vi "BRig_dataLC_Selection_PreR_Delay_l1.vi"() -> (2 "output_Selection_PreR_Delay":i32)   [LabVIEW 2014]
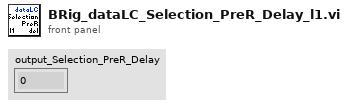
[diagram p1: front panel]
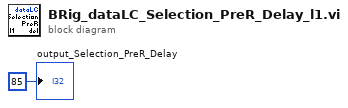
[diagram p0: block diagram]
diagram:
  "output_Selection_PreR_Delay" <- 85 ("output_iBlock")
